vi "oa_Check No Tacho Situation.vi"(7 "reset in":bool, 10 "speed profile":T1 {"speed [RPM]" format="%.2f"; "time [s]" format="%.2f"}, 11 "input duration":dbl) -> (5 "reset out":bool)   [LabVIEW 2017, in "SoundVib_TachProcess.lvlib"]
uses:
  <vilib>/addons/Sound and Vibration/Order Analysis/Tach Process/SoundVib_TachProcess.lvlib
  <vilib>/addons/Sound and Vibration/Order Analysis/Tach Process/SubVIs/speed profile.ctl
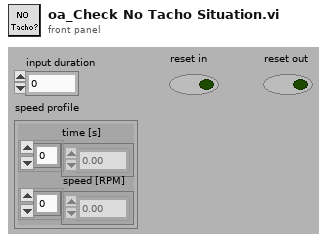
[diagram p1: front panel]
types:
  T1 = typedef "SoundVib_TachProcess.lvlib/speed profile.ctl" = cluster{"time [s]":dbl[], "speed [RPM]":dbl[]}
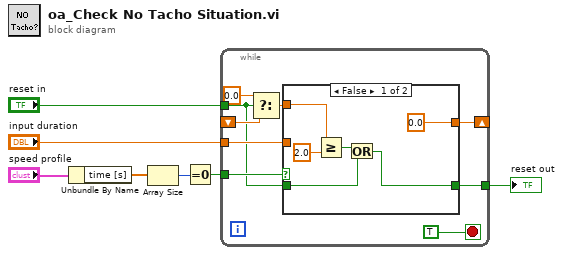
[diagram p0: block diagram]
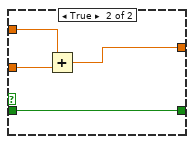
[diagram p2: hidden frame]
diagram:
  n1 = Unbundle By Name("speed profile") -> ("time [s]"=w6:dbl[])
  n2 = Array Size(array=w6) -> (size(s)=w5:i32)
  n3 = Equal To 0?(x=w5) -> (x = 0?=w4:bool)
  n4 = while {
    tunnel: w4 -> [w16]
    tunnel: "input duration" -> [w14]
    shift-right: [w13] -> _
    shift-left: _ -> [w12]
    tunnel: "reset in" -> [w9]
    tunnel: [w8] -> w1
    stop <- TRUE stop-if-true
    n5 = Select(t=0.0, s=w9, f=w12) -> (s? t:f=w10:dbl)
    n6 = case shown="False" w16 {
      tunnel: w14 -> [_ w26]
      tunnel: [0.0 w24] -> w13
      tunnel: w10 -> [w17 w25]
      tunnel: w9 -> [w19 w23]
      tunnel: [w18 w23] -> w8
      frame False {
        n7 = Greater Or Equal?(x=w17, y=2.0) -> (x >= y?=w20:bool)
        n8 = Or(x=w20, y=w19) -> (x .or. y?=w18:bool)
      }
      frame True {
        n9 = Add(x=w25, y=w26) -> (x+y=w24:dbl)
      }
    }
  }
  "reset out" <- w1
